vi "Controller Board Thermal Test.vi"(9 "Line in Voltage":dbl, 10 "Power Supply in":string, 11 "DMM in":string) -> (0 "error out":errorcluster, 3 "Temperature":dbl)   [LabVIEW 2025]
doc: "After applying maximum voltage and maximum ambient temperature, measure the temperature of the solar panel controller."
uses:
  Program Files (x86)/National Instruments/LabVIEW 2024/Instr.lib/Driver Simulation/Fixture/EnvironmentSettings.ctl
  Program Files (x86)/National Instruments/LabVIEW 2024/Instr.lib/Driver Simulation/Power Supply.lvlib
  Program Files (x86)/National Instruments/LabVIEW 2024/Instr.lib/Driver Simulation/DMM.lvlib
  Program Files (x86)/National Instruments/LabVIEW 2024/Instr.lib/Driver Simulation/Fixture.lvlib
  Program Files (x86)/National Instruments/LabVIEW 2024/Instr.lib/Driver Simulation/DMM/TemperatureSensorTypes.ctl
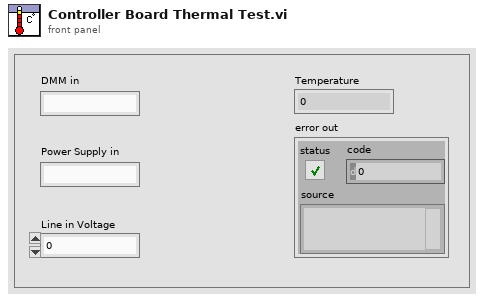
[diagram p1: front panel]
types:
  T1 = typedef "Driver Simulation.lvlib/Fixture.lvlib/EnvironmentSettings.ctl" = enum16{"Temperature", "Light Intensity"}
  T2 = typedef "Driver Simulation.lvlib/DMM.lvlib/TemperatureSensorTypes.ctl" = i32
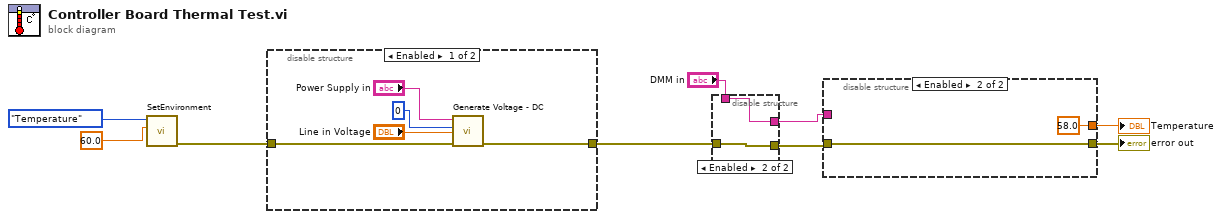
[diagram p0: block diagram]
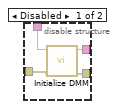
[diagram p2: hidden frame]
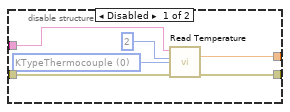
[diagram p4: hidden frame]
diagram:
  n1 = call "SetEnvironment.vi"("Value"=60.0, "Setting"=EnvironmentSettings."Temperature") -> ("error out"=w9:errorcluster)  [unwired: 9 in]
  n2 = disable-structure shown="Enabled" {
    disable-tunnel: w9 -> [w14 w15]
    disable-tunnel: [w10 w15] -> w4
    frame Enabled {
      n3 = call "Generate Voltage - DC.vi"("error in (no error)"=w14, "Output Voltage"="Line in Voltage", "Channel"=0, "Power Supply in"="Power Supply in") -> ("error out"=w10:errorcluster)  [unwired: 6 in, 1 out]
    }
    frame Disabled {
    }
  }
  n4 = disable-structure shown="Enabled" {
    disable-tunnel: w4 -> [w19 w21]
    disable-tunnel: [w18 w21] -> w3
    disable-tunnel: "DMM in" -> [w17 w20]
    disable-tunnel: [w16 w20] -> w1
    frame Disabled {
      n5 = call "Initialize DMM.vi"("error in (no error)"=w19, "DMM in"=w17) -> ("error out"=w18:errorcluster, "DMM out"=w16:string)  [unwired: 8 in]
    }
    frame Enabled {
    }
  }
  n6 = disable-structure shown="Enabled" {
    disable-tunnel: w3 -> [w27 w29]
    disable-tunnel: [w24 58.0 ("Temperature")] -> w6
    disable-tunnel: [w23 w29] -> w5
    disable-tunnel: w1 -> [w22 _]
    frame Disabled {
      w25 = T2 0 items=["KTypeThermocouple", "JTypeThermocouple"] ("Sensor Type")
      n7 = call "Read Temperature.vi"("error in (no error)"=w27, "Sensor Type"=w25, "Channel"=2, "DMM in"=w22) -> ("error out"=w23:errorcluster, "Temperature (C)"=w24:dbl)  [unwired: 5 in, 1 out]
    }
    frame Enabled {
    }
  }
  "Temperature" <- w6
  "error out" <- w5
